vi "Open gRPC Server-Client Code Generation VI.vi"   [LabVIEW 2019]
panel:
  # "Open gRPC Server-Client Code Generation VI..."
types:
  T1 = enum32{"Invalid", "Standard", "Closed", "Hidden", "Minimized", "Maximized"}
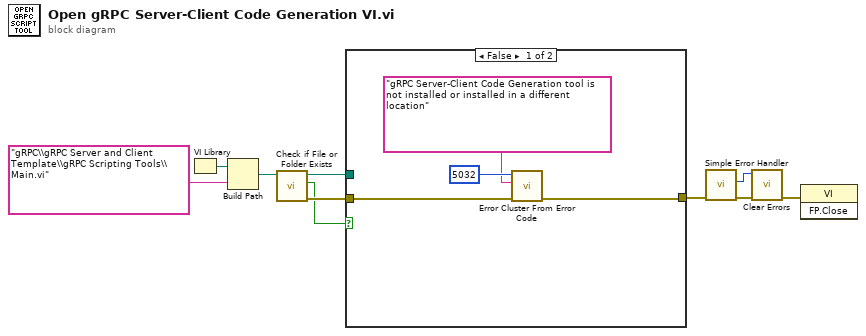
[diagram p0: block diagram]
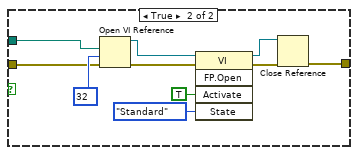
[diagram p2: hidden frame]
diagram:
  n1 = VI Library() -> (path=w10:path)
  n2 = Build Path(base path=w10, name or relative path="gRPC\\gRPC Server and Client Template\\gRPC Scripting Tools\\Main.vi") -> (appended path=w8:path)
  n3 = call <vilib>:"Check if File or Folder Exists.vi"("path"=w8) -> ("error out"=w7:errorcluster, "file or folder exists?"=w5:bool, "dup path"=w6:path)  [unwired: 8 in]
  n4 = case shown="False" w5 {
    tunnel: w7 -> [w14 w23]
    tunnel: w6 -> [_ w22]
    tunnel: [w13 w15] -> w4
    frame False {
      n5 = call <vilib>:"Error Cluster From Error Code.vi"("error in (no error)"=w14, "error message (\"\")"="gRPC Server-Client Code Generation tool is not installed or installed in a different location" ("error message (\"\")"), "error code (0)"=5032) -> ("error out"=w13:errorcluster)  [unwired: 6 in]
    }
    frame True {
      n6 = Open VI Reference(vi path=w22, options=32, error in (no error)=w23) -> (vi reference=w21:refnum<vi>, error out=w20:errorcluster)  [unwired: 3 in]
      n7 = invoke class="VI" method="FP.Open"(reference=w21, error in=w20, "Activate"=TRUE ("Activate?"), "State"=T1."Standard") -> (reference out=w16:refnum<vi>, error out=w17:errorcluster)  [unwired: 1 in, 3 out]
      n8 = Close Reference(reference=w16, error in (no error)=w17) -> (error out=w15:errorcluster)
    }
  }
  n9 = call <vilib>:"Simple Error Handler.vi"("error in (no error)"=w4) -> ("code out"=w2:i32, "error out"=w3:errorcluster)  [unwired: 4 in, 3 out]
  n10 = call <vilib>:"Clear Errors.vi"("error in (no error)"=w3, "specific error code to clear (0: all)"=w2) -> ("error out"=w1:errorcluster)  [unwired: 4 in, 1 out]
  n11 = invoke class="VI" method="FP.Close"(error in=w1) -> ()  [unwired: 2 in, 3 out]
